vi "Notify Of New Write.vi"(8 "error in":errorcluster, 11 "CIPC Reference":u64) -> (0 "error out":errorcluster)   [LabVIEW 2021, in "CIF_NI_CIPC.lvlib"]
doc: "Notify the CIPC readers which are waiting for new data. The function uses system calls so it should be avoided for maximum performance.s"
uses:
  CIF_NI_CIPC.lvlib
  <vilib>/Utility/error.llb/Trim Whitespace.vi
  <vilib>/Utility/error.llb/Error Cluster From Error Code.vi
  libnicipc.dll
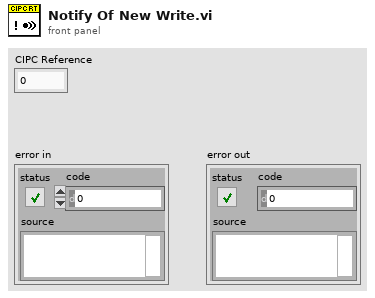
[diagram p1: front panel]
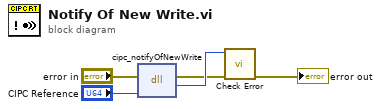
[diagram p0: block diagram]
diagram:
  n1 = dll-call lib="libnicipc.*" fn="cipc_notifyOfNewWrite"(error in="error in", "cipc_buffer_ref"="CIPC Reference") -> (error out=w4:errorcluster, "return type"=w5:i32)  [unwired: 3 in, 1 out]
  n2 = call "Check Error.vi"("error in (no error)"=w4, "Error Code"=w5) -> ("error out"=→"error out":errorcluster)  [unwired: 9 in]
